vi "Disconnection Siemens CPU.vi"(8 "error in (no error)":errorcluster, 11 "Siemens Ctr in":T1) -> (0 "error out":errorcluster, 3 "Siemens Ctr out":T1)   [LabVIEW 2014, in "Simatic S7.lvlib"]
uses:
  Simatic S7.lvlib
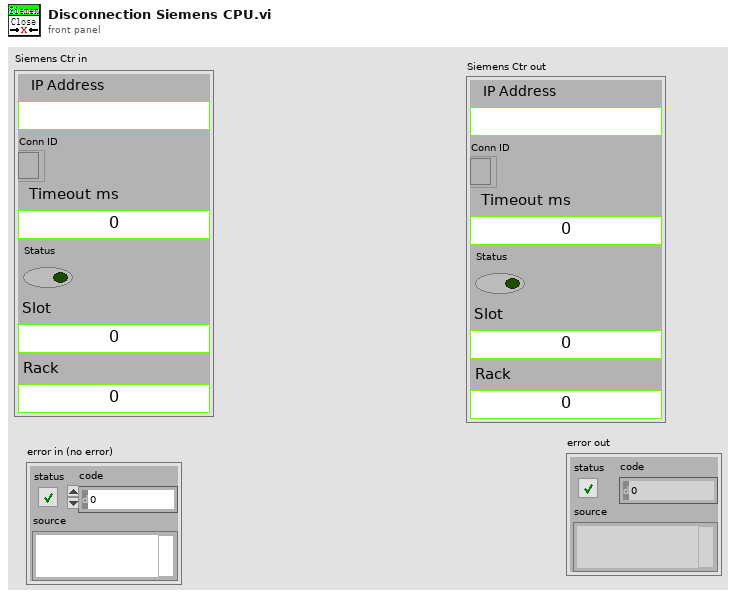
[diagram p1: front panel]
types:
  T1 = typedef "Simatic S7.lvlib/Siemens Ref.ctl" = cluster{"IP Address ":string, "Conn ID":refnum<k5>, "Timeout ms":i32, "Status":bool, "Slot":u16, "Rack":u16}
  T2 = typedef "Simatic S7.lvlib/Operation Siemens Ref.ctl" = enum16{"Init", "Add Ref", "Get Ref", "Set Error", "Close Close"}
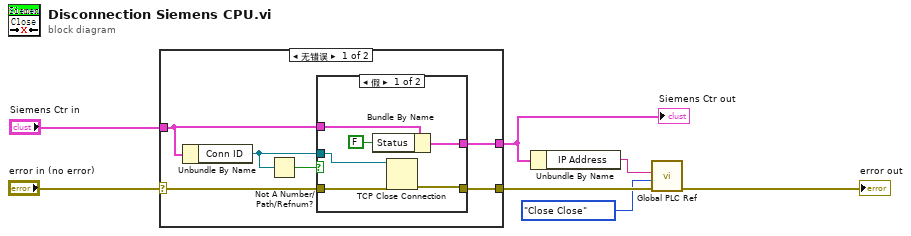
[diagram p0: block diagram]
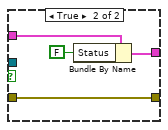
[diagram p2: hidden frame]
diagram:
  n1 = case shown="无错误" "error in (no error)" {
    selector: "error in (no error)" -> [w12 w24]
    tunnel: "Siemens Ctr in" -> [w10 w25]
    tunnel: [w9 w25] -> w3
    tunnel: [w8 w24] -> w5
    frame No Error {
      n2 = Unbundle By Name(w10) -> ("Conn ID"=w11:refnum<k5>)
      n3 = Not A Number/Path/Refnum?(number/path/refnum=w11) -> (NaN/Path/Refnum?=w13:bool)
      n4 = case shown="假" w13 {
        tunnel: w12 -> [w19 w20]
        tunnel: w11 -> [w18 _]
        tunnel: w10 -> [w17 w23]
        tunnel: [w15 w22] -> w9
        tunnel: [w14 w20] -> w8
        frame False {
          n5 = Bundle By Name(cluster=w17, "Status"=FALSE) -> (w15:T1)
          n6 = TCP Close Connection(connection ID=w18, error in (no error)=w19) -> (error out=w14:errorcluster)  [unwired: 1 in, 1 out]
        }
        frame True {
          n7 = Bundle By Name(cluster=w23, "Status"=FALSE) -> (w22:T1)
        }
      }
    }
    frame Error {
    }
  }
  "Siemens Ctr out" <- w3
  n8 = Unbundle By Name(w3) -> ("IP Address"=w2:string)
  n9 = call "Global PLC Ref.vi"("error in (no error)"=w5, "Operation Siemens Ref"=Operation_Siemens_Ref."Close Close", "IP Address"=w2) -> ("error out"=→"error out":errorcluster)  [unwired: 4 in, 4 out]
